vi "cgpa_sorter.vi"() -> ()   [LabVIEW 2014]
uses:
  <vilib>/Utility/file.llb/Read From Spreadsheet File (I64).vi
panel:
  out "sorted cgpa order":string[](array[string])
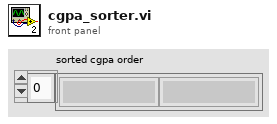
[diagram p1: front panel]
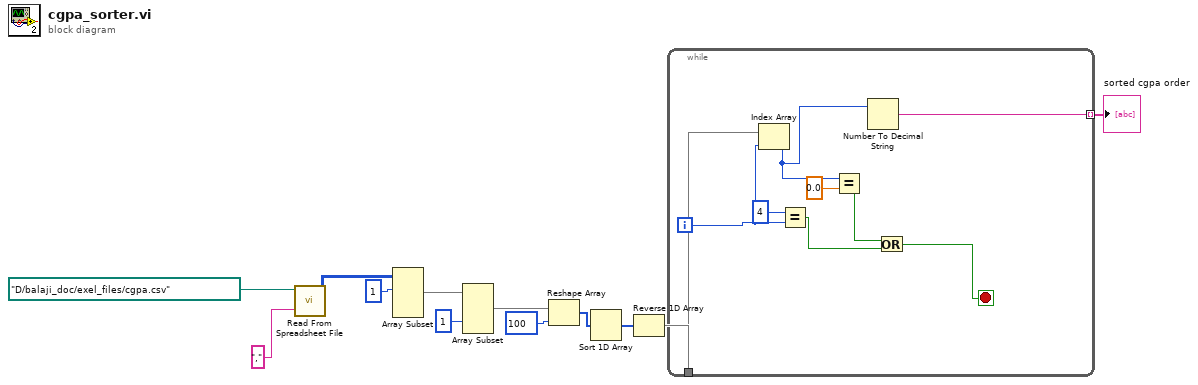
[diagram p0: block diagram]
diagram:
  n1 = call-poly <vilib>:"Read From Spreadsheet File.vi"("delimiter (\\t)"="," ("delimiter (\\t)"), "file path (dialog if empty)"=path "D:/balaji_doc/exel_files/cgpa.csv") -> ("all rows"=w8:i64[][])  [unwired: 5 in, 4 out]
  n2 = Array Subset(array=w8, index (row)=1 ("index")) -> (w10:i64[][])  [unwired: 3 in]
  n3 = Array Subset(array=w10, index (col)=1 ("index")) -> (w7:i64[][])  [unwired: 3 in]
  n4 = Reshape Array(w7, 100 ("dimension size")) -> (w5:i64[])
  n5 = Sort 1D Array(array=w5) -> (sorted array=w4:i64[])
  n6 = Reverse 1D Array(array=w4) -> (reversed array=w3:i64[])
  n7 = while {
    tunnel: w3 -> [w21]
    tunnel: [w13] -> w1 mode=indexing
    i -> [w19]
    stop <- w15 stop-if-true
    n8 = Index Array(array=w21, index=w19) -> (element=w14:i64)
    n9 = Equal?(x=4, y=w19) -> (x = y?=w17:bool)
    n10 = Equal?(x=w14, y=0.0) -> (x = y?=w16:bool)
    n11 = Number To Decimal String(number=w14) -> (decimal integer string=w13:string)  [unwired: 1 in]
    n12 = Or(x=w16, y=w17) -> (x .or. y?=w15:bool)
  }
  "sorted cgpa order" <- w1
